vi "NoSQLConn_Dialog.vi"() -> (0 "NewDSN":string, 1 "Boolean":bool, 2 "NewIPAddress":string)   [LabVIEW 2017]
panel:
  in  "OK Button":bool
  in  "OptionsSelector":u16(ring) items=["Load New Data Source Name", "Close the application"]
  # "System was not able to connect to the database...\nWhat do you want to do?"
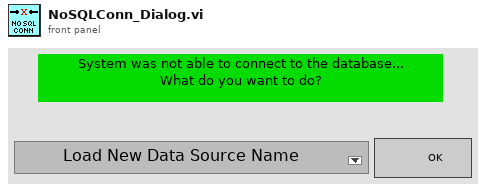
[diagram p1: front panel]
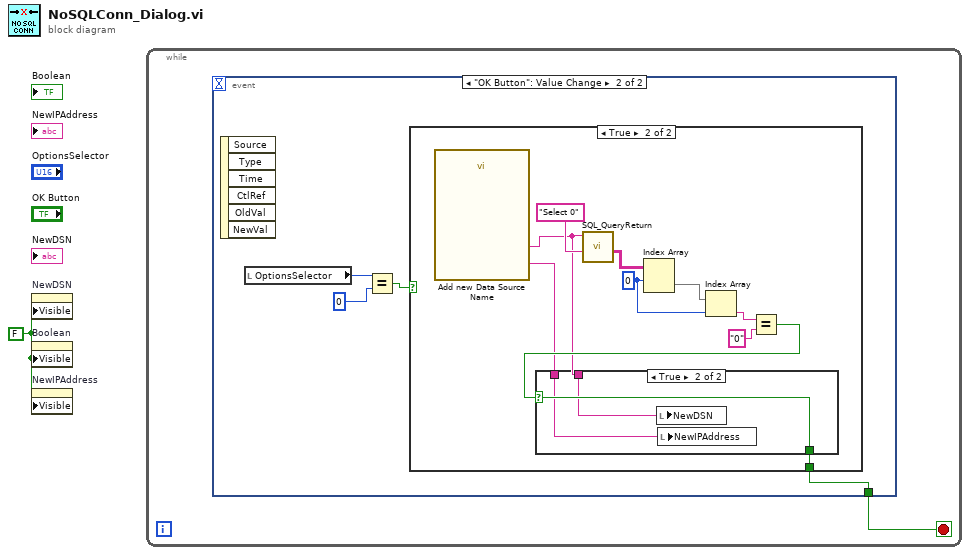
[diagram p0: block diagram]
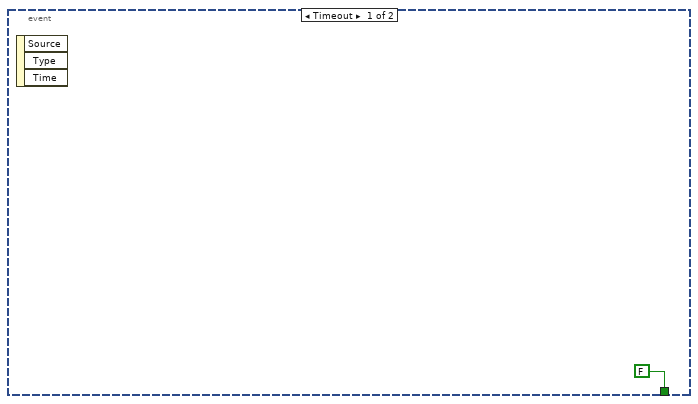
[diagram p2: hidden frame]
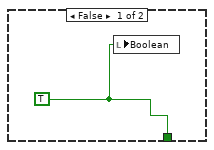
[diagram p3: hidden frame]
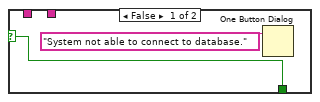
[diagram p4: hidden frame]
diagram:
  w1 = FALSE
  n1 = property on="NewDSN" class="Str"("Visible"=w1) -> ()  [unwired: 2 in, 2 out]
  n2 = property on="Boolean" class="Bool (strict)"("Visible"=w1) -> ()  [unwired: 2 in, 2 out]
  n3 = property on="NewIPAddress" class="Str"("Visible"=w1) -> ()  [unwired: 2 in, 2 out]
  n4 = while {
    stop <- w2 stop-if-true
    n5 = event shown="[1] \"OK Button\": Value Change" {
      selector: _ -> [_ _]
      dyn-events: _ -> [_ _]
      timeout: _ -> [_ _]
      tunnel: [FALSE w4] -> w2
      event Timeout {
        n6 = event-data() -> ()  [unwired: 1 in, 3 out]
      }
      event "OK Button": Value Change {
        n7 = event-data() -> ()  [unwired: 1 in, 6 out]
        n8 = local read "OptionsSelector"() -> (w7:u16)
        n9 = Equal?(x=w7, y=0) -> (x = y?=w5:bool)
        n10 = case shown="True" w5 {
          tunnel: [w8 w11] -> w4
          frame False {
            w8 = TRUE
            n11 = local write "Boolean"(w8) -> ()
          }
          frame True {
            w16 = 0 ("index (row)")
            n12 = call "Add new Data Source Name"() -> ("IP Address"=w9:string, "DSN"=w10:string)  [unwired: 16 in, 2 out]
            n13 = call "SQL_QueryReturn.vi"("SQL query"="Select 0", "ConnectionDSN"=w10) -> ("data"=w18:string[][])  [unwired: 9 in]
            n14 = Index Array(array=w18, index (row)=w16) -> (element=w17:string[])  [unwired: 1 in]
            n15 = Index Array(array=w17, index=w16) -> (element=w13:string)
            n16 = Equal?(x=w13, y="0" ("SQL query")) -> (x = y?=w12:bool)
            n17 = case shown="True" w12 {
              selector: w12 -> [w19 w23]
              tunnel: [w19 w23] -> w11
              tunnel: w10 -> [_ w22]
              tunnel: w9 -> [_ w21]
              frame False {
                n18 = One Button Dialog(message="System not able to connect to database." ("SQL query")) -> ()  [unwired: 1 in, 1 out]
              }
              frame True {
                n19 = local write "NewDSN"(w22) -> ()
                n20 = local write "NewIPAddress"(w21) -> ()
              }
            }
          }
        }
      }
    }
  }
